vi "Update Value.vi"(6 "Timestamp (Now)":dbl, 8 "error in (no error)":errorcluster, 9 "Raw Value (N/A)":dbl, 10 "Value":dbl, 11 "Channel in":refnum<class "Channel.lvclass">) -> (0 "error out":errorcluster, 3 "Channel out":refnum<class "Channel.lvclass">)   [LabVIEW 2020, in "Vecto.lvlib" / "Channel.lvclass"]
uses:
  Channel.lvclass
  Channel.lvclass/Channel.ctl
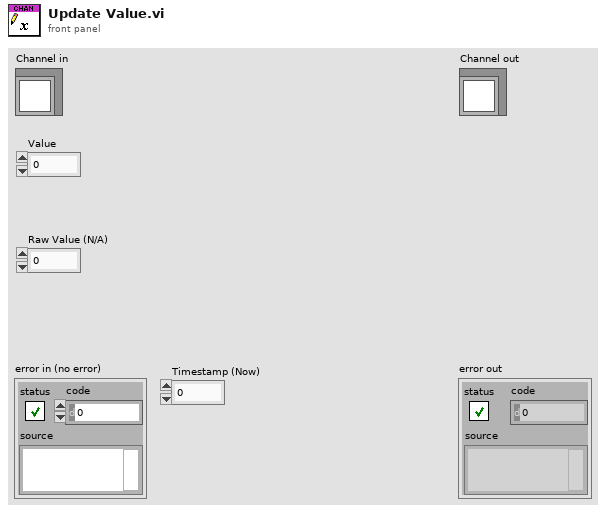
[diagram p1: front panel]
types:
  T1 = typedef "Vecto.lvlib/Channel.ctl" = cluster{"Info":T2, "Value":T3}
  T2 = typedef "Vecto.lvlib/Channel Info.ctl" = cluster{"Name":string, "Group":string, "Owning Node":u32, "Owning Task":u32, "Resource":string}
  T3 = typedef "Vecto.lvlib/Channel Value.ctl" = cluster{"Scaled":dbl, "Timestamp":dbl, "Raw":dbl}
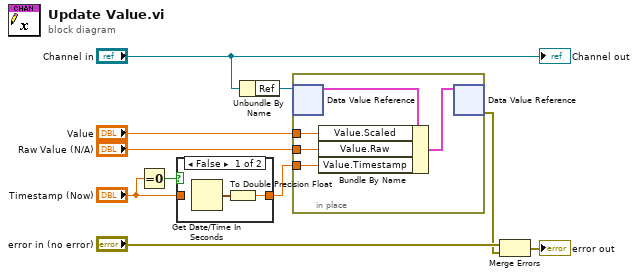
[diagram p0: block diagram]
diagram:
  n1 = Equal To 0?(x="Timestamp (Now)") -> (x = 0?=w5:bool)
  n2 = case shown="False" w5 {
    tunnel: "Timestamp (Now)" -> [_ w13]
    tunnel: [w11 w13] -> w3
    frame False {
      n3 = Get Date/Time In Seconds() -> (seconds since 1Jan1904=w12:timestamp)
      n4 = To Double Precision Float(number=w12) -> (double precision float=w11:dbl)
    }
    frame True {
    }
  }
  n5 = Unbundle By Name("Channel in") -> ("Ref"=w8:refnum<data-value>)
  n6 = in-place {
    in-place-border: "Value" -> [w17]
    in-place-border: "Raw Value (N/A)" -> [w16]
    in-place-border: w3 -> [w15]
    n7 = in-place-dvr #1(w8) -> (w18:T1)  [unwired: 1 out]
    n8 = Bundle By Name(cluster=w18, "Value.Scaled"=w17, "Value.Raw"=w16, "Value.Timestamp"=w15) -> (w14:T1)
    n9 = in-place-dvr #1(w14) -> (w1:errorcluster)  [unwired: 1 out]
  }
  n10 = Merge Errors("error in (no error)", w1) -> (→"error out":errorcluster)
  "Channel out" <- "Channel in"
